vi "SendRomiGyroProtocol.vi"(7 "Send":bool, 9 "Initialize":bool, 10 "Previous":T1={"type"="AI", "device"="", "name"="", "data"={"<init"=0, ">connected"=FALSE, "<offsetX"=0.0, "<offsetY"=0.0, "<offsetZ"=0.0, ">angle_x"=0.0, ">angle_y"=0.0, ">angle_z"=0.0, ">rate_x"=0.0, ">rate_y"=0.0, ">rate_z"=0.0, "<gain"=0.0}}, 11 "Current":T1={"type"="AI", "device"="", "name"="", "data"={"<init"=0, ">connected"=FALSE, "<offsetX"=0.0, "<offsetY"=0.0, "<offsetZ"=0.0, ">angle_x"=0.0, ">angle_y"=0.0, ">angle_z"=0.0, ">rate_x"=0.0, ">rate_y"=0.0, ">rate_z"=0.0, "<gain"=0.0}}) -> ()   [LabVIEW 2019]
uses:
  RomiGyro proto.ctl
  RomiGyro Data proto.ctl
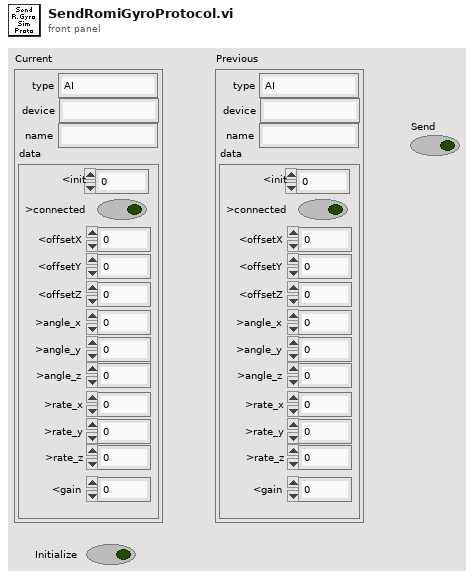
[diagram p1: front panel]
types:
  T1 = typedef "RomiGyro proto.ctl" = cluster{"type":string, "device":string, "name":string, "data":T2}
  T2 = typedef "RomiGyro Data proto.ctl" = cluster{"<init":i32, ">connected":bool, "<offsetX":dbl, "<offsetY":dbl, "<offsetZ":dbl, ">angle_x":dbl, ">angle_y":dbl, ">angle_z":dbl, ">rate_x":dbl, ">rate_y":dbl, ">rate_z":dbl, "<gain":dbl}
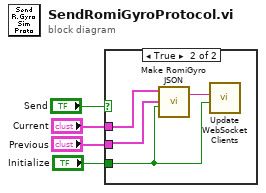
[diagram p0: block diagram]
diagram:
  n1 = case shown="True" "Send" {
    tunnel: "Current" -> [_ w8]
    tunnel: "Previous" -> [_ w7]
    tunnel: "Initialize" -> [_ w6]
    frame False {
    }
    frame True {
      n2 = call "Make RomiGyro JSON.vi"("Force"=w6, "Previous"=w7, "New"=w8) -> ("delta JSON"=w5:string)  [unwired: 8 in]
      n3 = call "Update WebSocket Clients.vi"("Initialize"=w6, "delta JSON"=w5) -> ()  [unwired: 10 in]
    }
  }
